vi "Forces.vi"() -> (3 "Forces":cluster{"Fy":dbl, "Fz":dbl, "Fx":dbl} {"Fy" format="%.1f"; "Fz" format="%.1f"; "Fx" format="%.1f"})   [LabVIEW 2019]
uses:
  <userlib>/HapticSTM/HapticSTM.lvlib
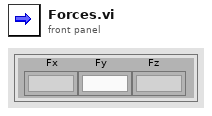
[diagram p1: front panel]
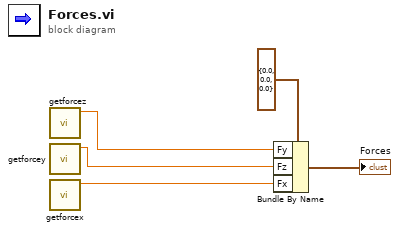
[diagram p0: block diagram]
diagram:
  n1 = call <userlib>:"getforcez.vi"() -> ("function return"=w1:dbl)  [unwired: 11 in]
  n2 = call <userlib>:"getforcey.vi"() -> ("function return"=w2:dbl)  [unwired: 11 in]
  n3 = call <userlib>:"getforcex.vi"() -> ("function return"=w3:dbl)  [unwired: 11 in]
  n4 = Bundle By Name(cluster=cluster{"Fy":dbl, "Fz":dbl, "Fx":dbl} {"Fy"=0.0, "Fz"=0.0, "Fx"=0.0} ("Forces"), "Fy"=w1, "Fz"=w2, "Fx"=w3) -> (→"Forces":cluster{"Fy":dbl, "Fz":dbl, "Fx":dbl})
